vi "Calculate Blob Info.vi"(0 "TypeDesc idx in":i32, 1 "Sub-desc size":i16, 5 "Blob size in":i16[](array[numeric]), 7 "Blob elem in":i16[](array[numeric]), 9 "Blob idx in":i16[](array[numeric]), 11 "Blob done in":bool[](array[boolean]), 12 "Blob dim":i16[](array[numeric])) -> (4 "TypeDesc idx out":i32, 6 "Blob size out":i16[](array[numeric]), 8 "Blob elem out":i16[](array[numeric]), 10 "Blob idx out":i16[](array[numeric]), 15 "Blob done out":bool[](array[boolean]))   [LabVIEW 2010]
doc: "See block diagram for VI documentation."
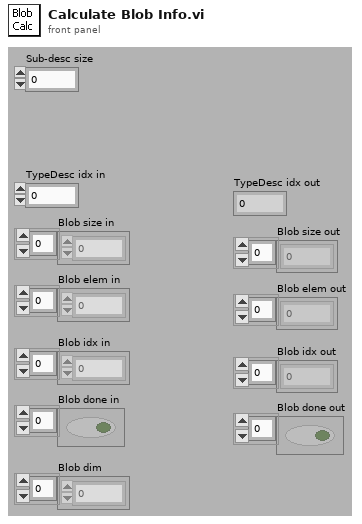
[diagram p1: front panel]
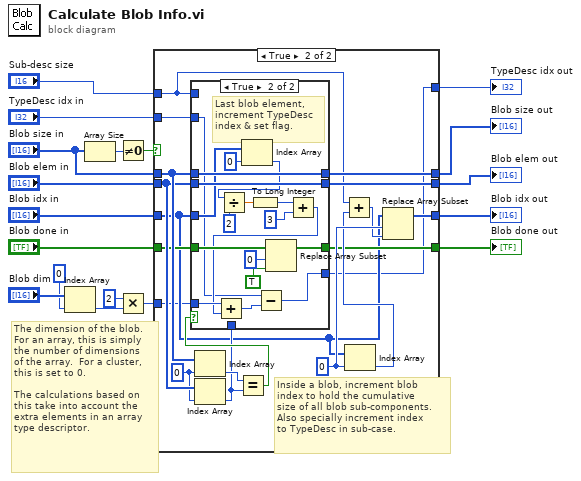
[diagram p0: block diagram]
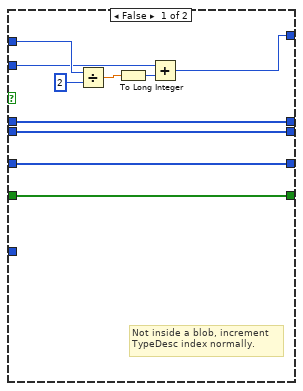
[diagram p2: hidden frame]
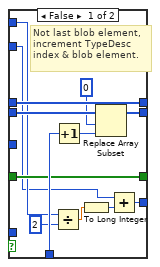
[diagram p3: hidden frame]
diagram:
  # "The dimension of the blob.\nFor an array, this is simply\nthe number of dimensions\nof the array.  For a cluster,\nthis is set to 0.\n\nThe calculations based on\nthis take into account the\nextra elements in an array\ntype descriptor."
  n1 = Index Array(array="Blob dim", index=0) -> (element=w3:i16)
  n2 = Array Size(array="Blob size in") -> (size(s)=w10:i32)
  n3 = Not Equal To 0?(x=w10) -> (x != 0?=w9:bool)
  n4 = Multiply(x=i16 2, y=w3) -> (x*y=w1:i16)
  n5 = case shown="True" w9 {
    tunnel: "Blob elem in" -> [w27 w46]
    tunnel: "Blob size in" -> [w28 w47]
    tunnel: [w28 w42] -> w13
    tunnel: [w27 w41] -> w14
    tunnel: "Blob idx in" -> [w26 w33]
    tunnel: "Blob done in" -> [w25 w35]
    tunnel: [w26 w39] -> w17
    tunnel: [w25 w34] -> w18
    tunnel: "TypeDesc idx in" -> [w19 w32]
    tunnel: "Sub-desc size" -> [w21 w31]
    tunnel: [w20 w30] -> w6
    tunnel: w1 -> [_ w29]
    frame False {
      # "Not inside a blob, increment\nTypeDesc index normally."
      n6 = Divide(x=w21, y=i16 2) -> (x/y=w24:dbl)
      n7 = To Long Integer(number=w24) -> (32bit integer=w23:i32)
      n8 = Add(x=w19, y=w23) -> (x+y=w20:i32)
    }
    frame True {
      w38 = 0 ("index")
      w45 = 0 ("index")
      # "Inside a blob, increment blob\nindex to hold the cumulative\nsize of all blob sub-components.\nAlso specially increment index\nto TypeDesc in sub-case."
      n9 = Index Array(array=w47, index=w45) -> (element=w43:i16)
      n10 = Index Array(array=w46, index=w45) -> (element=w40:i16)
      n11 = Equal?(x=w43, y=w40) -> (x = y?=w44:bool)
      n12 = case shown="True" w44 {
        tunnel: w47 -> [w60 w78]
        tunnel: w46 -> [w59 w77]
        tunnel: [w60 w78] -> w42
        tunnel: [w56 w77] -> w41
        tunnel: w40 -> [w58 _]
        tunnel: [w52 w75] -> w34
        tunnel: w35 -> [w52 w76]
        tunnel: [w53 w65] -> w30
        tunnel: w33 -> [_ w74]
        tunnel: w32 -> [w48 w61]
        tunnel: w31 -> [w49 _]
        tunnel: w29 -> [_ w64]
        frame False {
          # "Not last blob element,\nincrement TypeDesc\nindex & blob element."
          n13 = Divide(x=w49, y=i16 2) -> (x/y=w51:dbl)
          n14 = Increment(x=w58) -> (x+1=w57:i16)
          n15 = To Long Integer(number=w51) -> (32bit integer=w54:i32)
          n16 = Replace Array Subset(array=w59, new element=w57, index=0) -> (w56:i16[])
          n17 = Add(x=w48, y=w54) -> (x+y=w53:i32)
        }
        frame True {
          # "Last blob element,\nincrement TypeDesc\nindex & set flag."
          n18 = Index Array(array=w74, index=0) -> (element=w68:i16)
          n19 = Divide(x=w68, y=i16 2) -> (x/y=w73:dbl)
          n20 = To Long Integer(number=w73) -> (32bit integer=w72:i32)
          n21 = Replace Array Subset(array=w76, new element=TRUE ("new element/subarray"), index=0) -> (w75:bool[])
          n22 = Add(x=w72, y=3) -> (x+y=w63:i32)
          n23 = Add(x=w64, y=w63) -> (x+y=w62:i32)
          n24 = Subtract(x=w61, y=w62) -> (x-y=w65:i32)
        }
      }
      n25 = Index Array(array=w33, index=w38) -> (element=w36:i16)
      n26 = Add(x=w31, y=w36) -> (x+y=w37:i16)
      n27 = Replace Array Subset(array=w33, new element=w37, index=w38) -> (w39:i16[])
    }
  }
  "Blob done out" <- w18
  "Blob idx out" <- w17
  "TypeDesc idx out" <- w6
  "Blob elem out" <- w14
  "Blob size out" <- w13
